vi "GetIncreasingStartegy.vi"(2 "error in (no error)":errorcluster, 4 "VISA resource name":refnum<visa-resource-name>) -> (0 "error out":errorcluster, 1 "VISA resource name out":refnum<visa-resource-name>, 3 "Sample Increasing Startegy":u16(ring) items=["Interpolation", "Return Zero", "Hold Last", "Samples Duplication"])   [LabVIEW 2020, in "Active Technologies AWG3000.lvlib"]
uses:
  Active Technologies AWG3000.lvlib
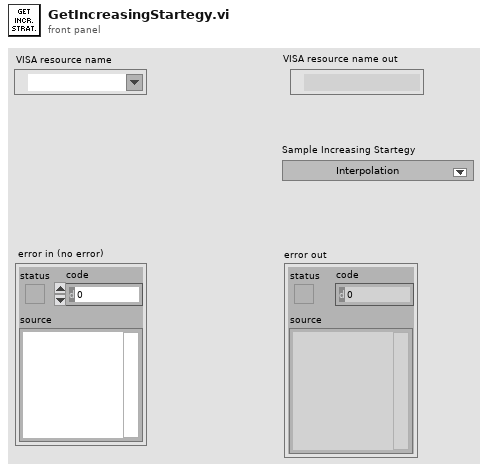
[diagram p1: front panel]
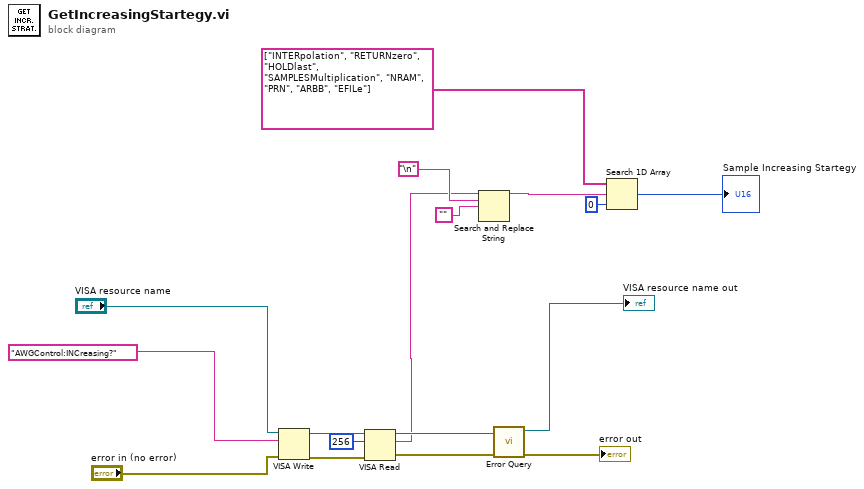
[diagram p0: block diagram]
diagram:
  n1 = VISA Write(VISA resource name="VISA resource name", write buffer="AWGControl:INCreasing?", error in (no error)="error in (no error)") -> (VISA resource name out=w15:refnum<visa-resource-name>, error out=w14:errorcluster)  [unwired: 1 out]
  n2 = VISA Read(VISA resource name=w15, byte count=u32 256, error in (no error)=w14) -> (VISA resource name out=w12:refnum<visa-resource-name>, read buffer=w3:string, error out=w11:errorcluster)  [unwired: 1 out]
  n3 = Search and Replace String(input string=w3, search string="\n", replace string="") -> (result string=w4:string)  [unwired: 5 in, 3 out]
  n4 = call "Error Query.vi"("error in (no error)"=w11, "VISA resource name"=w12) -> ("error out"=→"error out":errorcluster, "VISA resource name out"=→"VISA resource name out":refnum<visa-resource-name>)  [unwired: 6 in, 2 out]
  n5 = Search 1D Array(1D array=string[] ["INTERpolation", "RETURNzero", "HOLDlast", "SAMPLESMultiplication", "NRAM", "PRN", "ARBB", "EFILe"], element=w4, start index (0)=0) -> (index of element=→"Sample Increasing Startegy":i32)
